vi "Advance past whitespace.vi"(4 "Past Colon":bool, 6 "Past Comma":bool, 7 "JSON":string, 9 "Offset":i32, 11 "Parser State in":T1=enum."Leading Whitespace") -> (0 "Comma Not Found":bool, 1 "Offset of first non-whitespace":i32, 3 "Parser State":T1)   [LabVIEW 2020, in "JSONtext.lvlib"]
uses:
  <vilib>/JDP Science/JSONtext/JSONtext.lvlib
  <vilib>/JDP Science/JSONtext/Parsing/Parsing State.ctl
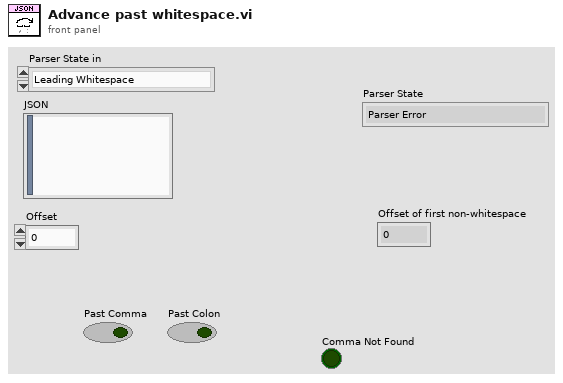
[diagram p1: front panel]
types:
  T1 = typedef "JSONtext.lvlib/Parsing State.ctl" = enum16{"Parser Error", "Object", "Array", "String", "Number/Other", "Leading Whitespace", "Object end", "Array end", "Value end"}
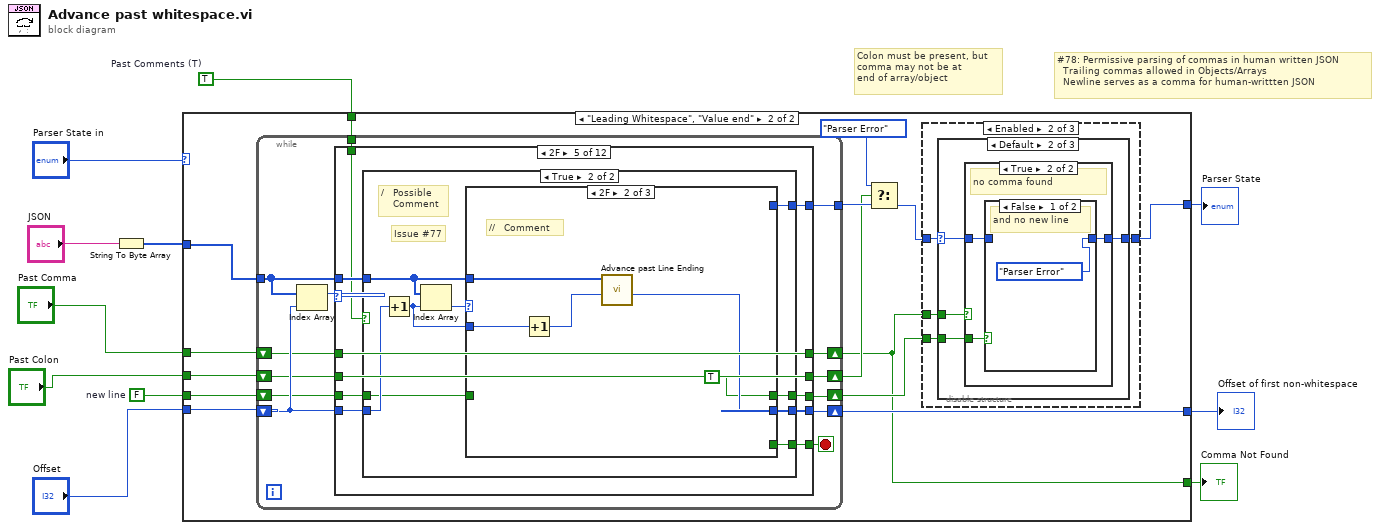
[diagram p0: block diagram]
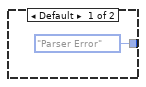
[diagram p5: hidden frame]
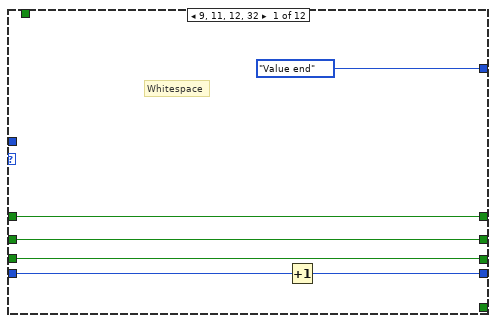
[diagram p11: hidden frame]
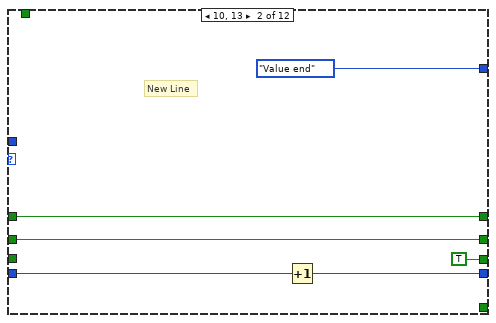
[diagram p12: hidden frame]
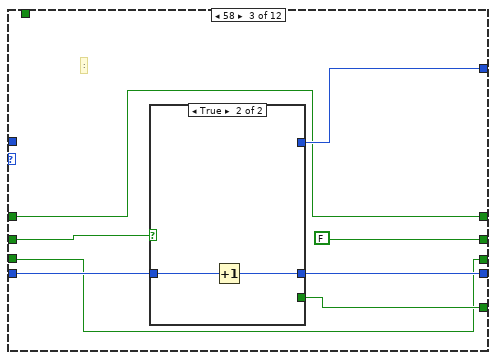
[diagram p13: hidden frame]
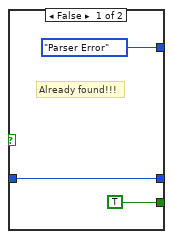
[diagram p14: hidden frame]
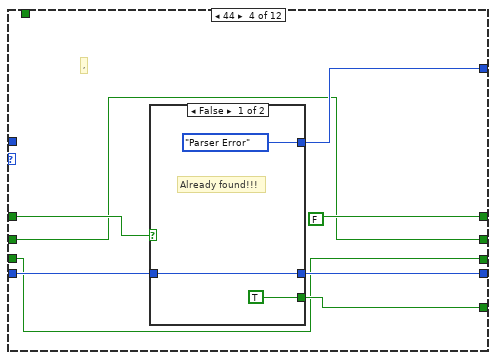
[diagram p15: hidden frame]
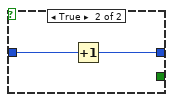
[diagram p16: hidden frame]
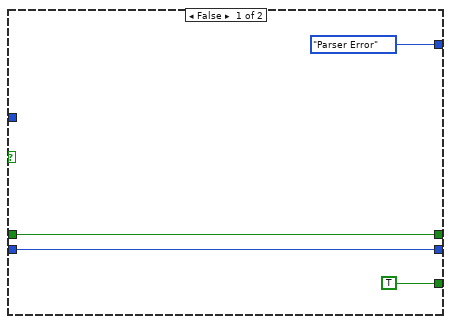
[diagram p17: hidden frame]
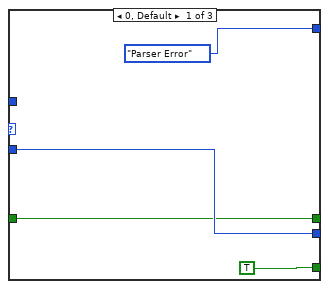
[diagram p18: hidden frame]
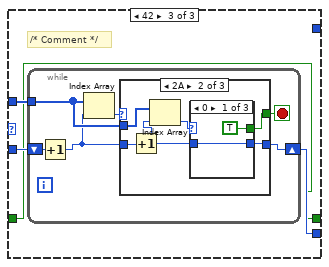
[diagram p19: hidden frame]
diagram:
  w2 = FALSE  # new line
  w3 = TRUE  # Past Comments (T)
  # "#78: Permissive parsing of commas in human written JSON\n  Trailing commas allowed in Objects/Arrays\n  Newline serves as a comma for human-writtten JSON"
  # "Colon must be present, but\ncomma may not be at\nend of array/object"
  n1 = String To Byte Array(string="JSON") -> (unsigned byte array=w5:u8[])
  n2 = case shown="\"Leading Whitespace\", \"Value end\"" "Parser State in" {
    selector: "Parser State in" -> [w13 _]
    tunnel: [w13 w27] -> w11
    tunnel: [w12 w26] -> w10
    tunnel: "Offset" -> [w12 w25]
    tunnel: w5 -> [_ w18]
    tunnel: "Past Comma" -> [_ w24]
    tunnel: "Past Colon" -> [_ w23]
    tunnel: w3 -> [_ w17]
    tunnel: w2 -> [_ w16]
    tunnel: [_ w14] -> w1
    frame "Parser Error", Default {
    }
    frame "Leading Whitespace", "Value end" {
      n3 = while {
        tunnel: w18 -> [w55]
        shift-right: [w60] -> w26
        shift-left: w25 -> [w61]
        tunnel: [w63] -> w22
        shift-right: [w59] -> w14
        shift-left: w24 -> [w58]
        shift-right: [w56] -> w20
        shift-left: w23 -> [w57]
        tunnel: w17 -> [w54]
        shift-right: [w52] -> w15
        shift-left: w16 -> [w53]
        stop <- w62 stop-if-true
        n4 = Index Array(array=w55, index=w61) -> (element=w64:u8)
        n5 = case shown="2F" w64 {
          tunnel: [Parsing_State."Value end" Parsing_State."Value end" w82 w95 w107 Parsing_State."String" Parsing_State."Number/Other" Parsing_State."Array" Parsing_State."Array end" Parsing_State."Object" Parsing_State."Object end" Parsing_State."Parser Error"] -> w63
          tunnel: [_ _ w81 w94 w106 TRUE TRUE TRUE TRUE TRUE TRUE TRUE] -> w62
          tunnel: w61 -> [w70 w76 w84 w97 w110 w164 w170 w176 w182 w188 w194 w202]
          tunnel: [w69 w75 w83 w96 w108 w164 w170 w176 w182 w188 w194 w202] -> w60
          tunnel: [w67 w73 w78 FALSE ("Allow Comma") w112 w163 w169 w175 w181 w187 w193 w199] -> w59
          tunnel: w58 -> [w67 w73 w78 w93 w112 w163 w169 w175 w181 w187 w193 w199]
          tunnel: [w66 w72 FALSE ("Allow Comma") w91 w111 w162 w168 w174 w180 w186 w192 w198] -> w56
          tunnel: w57 -> [w66 w72 w80 w91 w111 w162 w168 w174 w180 w186 w192 w198]
          tunnel: w55 -> [_ _ _ _ w109 _ _ _ _ _ _ _]
          tunnel: w54 -> [_ _ _ _ w105 _ _ _ _ _ _ _]
          tunnel: w53 -> [w65 _ w77 w90 w104 w161 w167 w173 w179 w185 w191 w197]
          tunnel: [w65 TRUE w77 w90 w103 w161 w167 w173 w179 w185 w191 w197] -> w52
          frame 9, 11, 12, 32 {
            # "Whitespace"
            n6 = Increment(x=w70) -> (x+1=w69:i32)
          }
          frame 10, 13 {
            # "New Line"
            n7 = Increment(x=w76) -> (x+1=w75:i32)
          }
          frame 58 {
            # ":"
            n8 = case shown="True" w80 {
              tunnel: w84 -> [w86 w89]
              tunnel: [w86 w88] -> w83
              tunnel: [Parsing_State."Parser Error" _] -> w82
              tunnel: [TRUE _] -> w81
              frame False {
                # "Already found!!!"
              }
              frame True {
                n9 = Increment(x=w89) -> (x+1=w88:i32)
              }
            }
          }
          frame 44 {
            # ","
            n10 = case shown="False" w93 {
              tunnel: w97 -> [w99 w102]
              tunnel: [w99 w101] -> w96
              tunnel: [Parsing_State."Parser Error" _] -> w95
              tunnel: [TRUE _] -> w94
              frame False {
                # "Already found!!!"
              }
              frame True {
                n11 = Increment(x=w102) -> (x+1=w101:i32)
              }
            }
          }
          frame 47 {
            n12 = case shown="True" w105 {
              tunnel: w110 -> [w115 w125]
              tunnel: w109 -> [_ w123]
              tunnel: [w115 w121] -> w108
              tunnel: [Parsing_State."Parser Error" ("t") w120] -> w107
              tunnel: [TRUE w119] -> w106
              tunnel: w104 -> [w113 w118]
              tunnel: [w113 w117] -> w103
              frame False {
              }
              frame True {
                # "Issue #77"
                # "/   Possible \n    Comment"
                n13 = Increment(x=w125) -> (x+1=w122:i32)
                n14 = Index Array(array=w123, index=w122) -> (element=w124:u8)
                n15 = case shown="2F" w124 {
                  tunnel: w123 -> [_ w134 w138]
                  tunnel: w122 -> [w127 w133 w136]
                  tunnel: [w127 w132 w137] -> w121
                  tunnel: [Parsing_State."Parser Error" ("t") _ _] -> w120
                  tunnel: [TRUE _ _] -> w119
                  tunnel: w118 -> [w126 _ w135]
                  tunnel: [w126 TRUE w135] -> w117
                  frame 0, Default {
                  }
                  frame 47 {
                    # "//   Comment"
                    n16 = Increment(x=w133) -> (x+1=w131:i32)
                    n17 = call <vilib>:"Advance past Line Ending.vi"("Offset"=w131, "JSON"=w134) -> ("Offset after Line Ending"=w132:i32)  [unwired: 9 in]
                  }
                  frame 42 {
                    # "/* Comment */"
                    n18 = while {
                      tunnel: w138 -> [w141]
                      shift-right: [w142] -> w137
                      shift-left: w136 -> [w140]
                      stop <- w143 stop-if-true
                      n19 = Increment(x=w140) -> (x+1=w139:i32)
                      n20 = Index Array(array=w141, index=w139) -> (element=w144:u8)
                      n21 = case shown="2A" w144 {
                        tunnel: w139 -> [w145 w149 w160]
                        tunnel: [_ w146 TRUE] -> w143
                        tunnel: [w145 w147 w160] -> w142
                        tunnel: w141 -> [_ w148 _]
                        frame Default {
                        }
                        frame 42 {
                          n22 = Increment(x=w149) -> (x+1=w150:i32)
                          n23 = Index Array(array=w148, index=w150) -> (element=w151:u8)
                          n24 = case shown="0" w151 {
                            tunnel: [TRUE FALSE TRUE] -> w146
                            tunnel: w150 -> [w153 w155 w157]
                            tunnel: [w153 w155 w156] -> w147
                            frame 0 {
                            }
                            frame Default {
                            }
                            frame 47 {
                              n25 = Increment(x=w157) -> (x+1=w156:i32)
                            }
                          }
                        }
                        frame 0 {
                        }
                      }
                    }
                  }
                }
              }
            }
          }
          frame 34 {
          }
          frame 43, 45, 46, 48..57, 69, 73, 78, 101, 102, 110, 116 {
          }
          frame 91 {
          }
          frame 93 {
          }
          frame 123 {
          }
          frame 125 {
          }
          frame Default {
          }
        }
      }
      n26 = Select(t=Parsing_State."Parser Error", s=w20, f=w22) -> (s? t:f=w19:T1)
      n27 = disable-structure shown="Enabled" {
        disable-tunnel: [w30 w39 _] -> w27
        disable-tunnel: w14 -> [w29 w38 _]
        disable-tunnel: w19 -> [w28 w37 _]
        disable-tunnel: w15 -> [_ w36 _]
        frame Disabled {
          n28 = case shown="True" w29 {
            tunnel: w28 -> [w31 w33]
            tunnel: [w31 w32] -> w30
            frame False {
            }
            frame True {
              # "Comma not found is OK\nonly if Object or Array end"
              n29 = case shown="\"Object end\", \"Array end\"" w33 {
                selector: w33 -> [_ w35]
                tunnel: [Parsing_State."Parser Error" w35] -> w32
                frame Default {
                }
                frame "Object end", "Array end" {
                }
              }
            }
          }
        }
        frame Enabled {
          n30 = case shown="Default" w37 {
            selector: w37 -> [w40 w42 w51]
            tunnel: [w40 w43 w51] -> w39
            tunnel: w38 -> [_ w44 _]
            tunnel: w36 -> [_ w41 _]
            frame "Parser Error" {
            }
            frame Default {
              n31 = case shown="True" w44 {
                tunnel: [w45 w46] -> w43
                tunnel: w42 -> [w45 w47]
                tunnel: w41 -> [_ w48]
                frame False {
                }
                frame True {
                  # "no comma found"
                  n32 = case shown="False" w48 {
                    tunnel: w47 -> [_ w50]
                    tunnel: [Parsing_State."Parser Error" ("t") w50] -> w46
                    frame False {
                      # "and no new line"
                    }
                    frame True {
                      # "Counts as a\ncomma"
                      # "but new line"
                    }
                  }
                }
              }
            }
            frame "Object end", "Array end" {
              # "At Object or Array end\nwe usually have no comma\nbut accept a comma"
            }
          }
        }
        frame Disabled {
        }
      }
    }
  }
  "Parser State" <- w11
  "Offset of first non-whitespace" <- w10
  "Comma Not Found" <- w1
